vi "Read data type.vi"(8 "error in (no error)":errorcluster, 11 "Class 2 in":refnum<class "Class 2345678.lvclass">) -> (0 "error out":errorcluster, 2 "data type":T1, 3 "Class 2 out":refnum<class "Class 2345678.lvclass">)   [LabVIEW 2016, in "Data Sharing Framework.Runtime.lvlib" / "Class 2345678.lvclass"]
uses:
  Class 2345678.lvclass
  <vilib>/NI Veristand/VeriStand Data/Typedefs/Typedefs.Data Types.ctl
  Class 2345678.lvclass/Class 2345678.ctl
  <vilib>/NI Veristand/VeriStand Data/VeriStand Data.lvlib
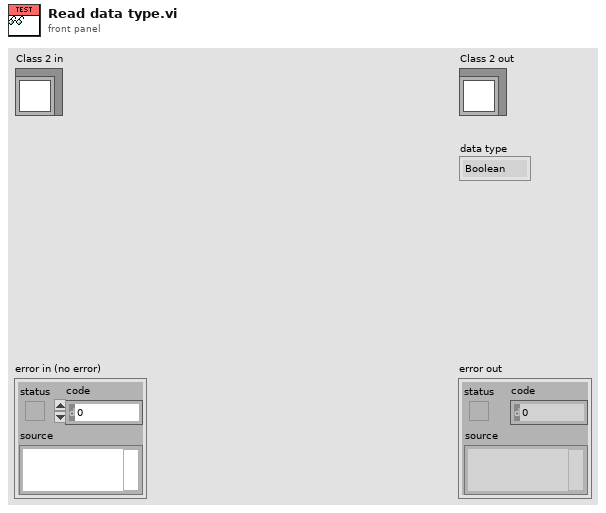
[diagram p1: front panel]
types:
  T1 = typedef "VeriStand Data.lvlib/Typedefs.Data Types.ctl" = enum16{"Boolean", "Single", "Double", "I8", "I16", "I32", "I64", "U8", "U16", "U32", "U64"}
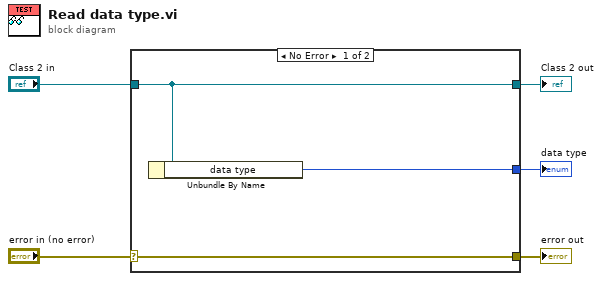
[diagram p0: block diagram]
diagram:
  n1 = case shown="No Error" "error in (no error)" {
    selector: "error in (no error)" -> [w8 w9]
    tunnel: [w8 w9] -> w4
    tunnel: [w7 w10] -> w2
    tunnel: "Class 2 in" -> [w7 w10]
    tunnel: [w6 _] -> w1
    frame No Error {
      n2 = Unbundle By Name(w7) -> ("data type"=w6:T1)
    }
    frame Error {
    }
  }
  "error out" <- w4
  "Class 2 out" <- w2
  "data type" <- w1
